vi "SaveBmpToFile.vi"(8 "error in (no error)":errorcluster caption="错误输入（无错误）", 9 "文件格式":T1(ring), 10 "路径":path, 11 "Screen 输入":refnum<class "Screen.lvclass"> caption="DNL_LabVIEW Object in") -> (0 "error out":errorcluster caption="错误输出", 3 "Screen 输出":refnum<class "Screen.lvclass"> caption="DNL_LabVIEW Object out")   [LabVIEW 2011, in "Screen.lvclass"]
uses:
  Screen.lvclass
  Screen.lvclass/Screen.ctl
  System.Drawing
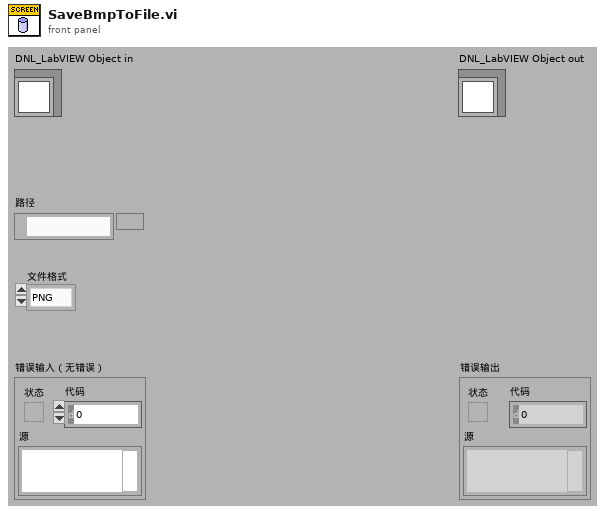
[diagram p1: front panel]
types:
  T1 = enum16{"PNG", "TIFF", "EMF", "JPEG", "BMP", "GIF"}
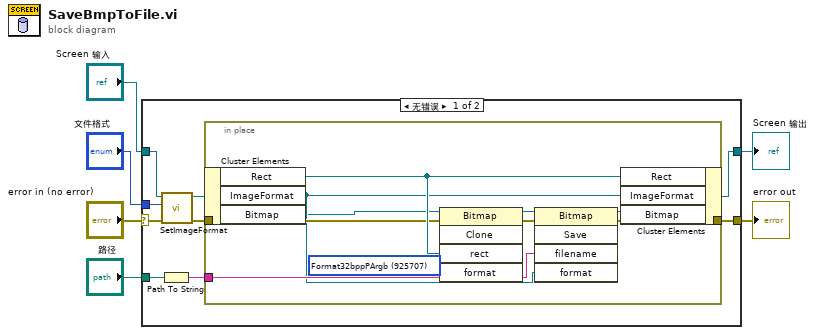
[diagram p0: block diagram]
diagram:
  n1 = case shown="无错误" "error in (no error)" {
    selector: "error in (no error)" -> [w13 w27]
    tunnel: [w9 w27] -> w5
    tunnel: [w10 w26] -> w4
    tunnel: "Screen 输入" -> [w14 w26]
    tunnel: "文件格式" -> [w15 _]
    tunnel: "路径" -> [w8 _]
    frame No Error {
      n2 = Path To String(path=w8) -> (string=w7:string)
      n3 = call "SetImageFormat.vi"("error in (no error)"=w13, "文件格式"=w15, "Screen 输入"=w14) -> ("error out"=w11:errorcluster, "Screen 输出"=w12:refnum<class "Screen.lvclass">)  [unwired: 7 in]
      n4 = in-place {
        in-place-border: w11 -> [w21]
        in-place-border: [w20] -> w9
        in-place-border: w7 -> [w19]
        w25 = 925707 items=["DontCare, Undefined"=0, "Max"=15, "Indexed"=65536, "Gdi"=131072, "Format16bppRgb555"=135173, "Format16bppRgb565"=135174, "Format24bppRgb"=137224, "Format32bppRgb"=139273, "Format1bppIndexed"=196865, "Format4bppIndexed"=197634, "Format8bppIndexed"=198659, "Alpha"=262144, "Format16bppArgb1555"=397319, "PAlpha"=524288, "Format32bppPArgb"=925707, "Extended"=1048576, "Format16bppGrayScale"=1052676, "Format48bppRgb"=1060876, "Format64bppPArgb"=1851406, "Canonical"=2097152, "Format32bppArgb"=2498570, "Format64bppArgb"=3424269] ("format")
        n5 = in-place-cluster #1(w12) -> ("Rect"=w24:refnum<k24>, "ImageFormat"=w18:refnum<k24>, "Bitmap"=w17:refnum<k24>)
        n6 = invoke class="Bitmap" method="Clone"(reference=w17, error in=w21, "rect"=w24, "format"=w25) -> (reference out=w23:refnum<k24>, error out=w22:errorcluster)  [unwired: 1 in, 3 out]
        n7 = invoke class="Bitmap" method="Save"(reference=w23, error in=w22, "filename"=w19, "format"=w18) -> (reference out=w16:refnum<k24>, error out=w20:errorcluster)  [unwired: 1 in, 3 out]
        n8 = in-place-cluster #1("Rect"=w24, "ImageFormat"=w18, "Bitmap"=w16) -> (w10:refnum<class "Screen.lvclass">)
      }
    }
    frame Error {
    }
  }
  "error out" <- w5
  "Screen 输出" <- w4
